vi "Incremental Servo (SubVI).vi"(6 "error in (no error)":errorcluster, 7 "Threshold":dbl, 8 "Axis Value":dbl, 9 "Servo refnum":string="My Servo RefNum") -> (0 "error out":errorcluster)   [LabVIEW 2013]
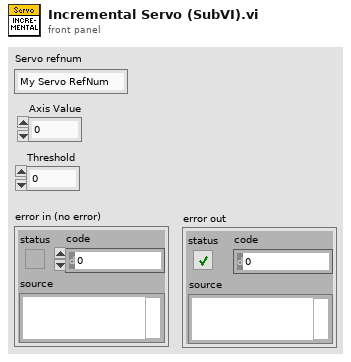
[diagram p1: front panel]
types:
  T1 = typedef "WPI_ServoDeviceRef.ctl" = cluster{"DeviceStatus":errorcluster, "Digital Module":T2, "PWM Channel":T3, "DeadBand":T4}
  T2 = typedef "FPGA_TypedefDigitalModule.ctl" = enum16{"Digital Module 1", "Digital Module 2"}
  T3 = typedef "FPGA_DIOPWMChannel.ctl" = enum8{"PWM 1", "PWM 2", "PWM 3", "PWM 4", "PWM 5", "PWM 6", "PWM 7", "PWM 8", "PWM 9", "PWM 10", "Invalid"}
  T4 = typedef "WPI_PWMDeadband.ctl" = cluster{"Name":string, "maxPositivePwm":i32, "minPositivePwm":i32, "centerPwm":i32, "maxNegativePwm":i32, "minNegativePwm":i32, "angularRange":u16}
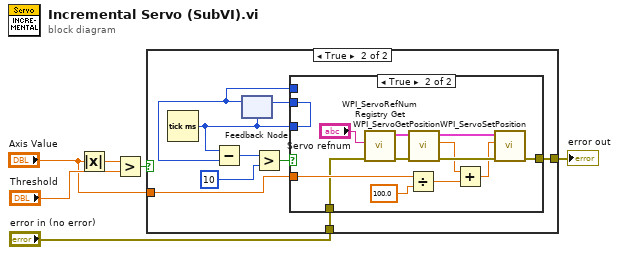
[diagram p0: block diagram]
diagram:
  n1 = Absolute Value(x="Axis Value") -> (abs(x)=w2:dbl)
  n2 = Greater?(x=w2, y="Threshold") -> (0:w6:bool)
  n3 = case shown="True" w6 {
    tunnel: "Axis Value" -> [_ w14]
    tunnel: "error in (no error)" -> [w7 w9]
    tunnel: [w7 w8] -> w3
    frame False {
    }
    frame True {
      n4 = Tick Count (ms)() -> (millisecond timer value=w12:u32)
      n5 = feedback #1(w12) -> (w11:u32)
      n6 = Subtract(x=w12, y=w11) -> (x-y=w15:u32)
      n7 = Greater?(x=w15, y=u32 10 ("x")) -> (0:w16:bool)
      n8 = case shown="True" w16 {
        tunnel: w14 -> [_ w28]
        tunnel: w11 -> [w18 _]
        tunnel: w12 -> [_ w26]
        tunnel: [w18 w26] -> w13
        tunnel: w9 -> [w17 w21]
        tunnel: [w17 w20] -> w8
        frame False {
        }
        frame True {
          n9 = call <vilib>:"WPI_ServoRefNum Registry Get.vi"("error in (no error)"=w21, "refnum name"="Servo refnum") -> ("error out"=w22:errorcluster, "ServoDeviceRef"=w31:T1)  [unwired: 8 in]
          n10 = Divide(x=w28, y=100.0) -> (x/y=w29:dbl)
          n11 = call <vilib>:"WPI_ServoGetPosition.vi"("error in (no error)"=w22, "ServoDeviceRef"=w31) -> ("error out"=w25:errorcluster, "Position"=w23:dbl, "ServoDeviceRef"=w30:T1)  [unwired: 7 in]
          n12 = Add(x=w23, y=w29) -> (x+y=w24:dbl)
          n13 = call <vilib>:"WPI_ServoSetPosition.vi"("error in (no error)"=w25, "Position"=w24, "ServoDeviceRef"=w30) -> ("error out"=w20:errorcluster)  [unwired: 7 in, 1 out]
        }
      }
      n14 = feedback-in #1(w13) -> ()
    }
  }
  "error out" <- w3
